vi "http 400 bad request.vi"(11 "application request in":T4) -> (3 "application request out":T1)   [LabVIEW 2016, in "Basic HTTP server.lvclass"]
uses:
  Basic HTTP server.lvclass
  http request.ctl
  http method.ctl
  HTTP headers/http header data.ctl
  http response.ctl
  http response packet type.ctl
  HTTP headers/http headers.lvlib
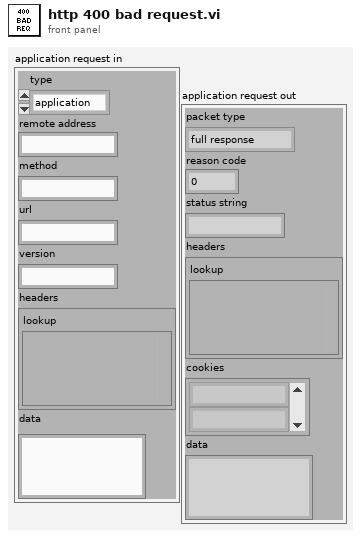
[diagram p1: front panel]
types:
  T1 = typedef "Basic HTTP server.lvclass/http response.ctl" = cluster{"packet type":T2, "reason code":u16, "status string":string, "headers":T3, "cookies":string[], "data":string}
  T2 = typedef "Basic HTTP server.lvclass/http response packet type.ctl" = enum16{"full response", "header only", "data only", "last data", "raw output"}
  T3 = typedef "http headers.lvlib/http header data.ctl" = cluster{"lookup":variant}
  T4 = typedef "Basic HTTP server.lvclass/http request.ctl" = cluster{"type":T5, "remote address":string, "method":string, "url":string, "version":string, "headers":T3, "data":string}
  T5 = typedef "Basic HTTP server.lvclass/http method.ctl" = enum16{"application", "error", "upgrade", "expect"}
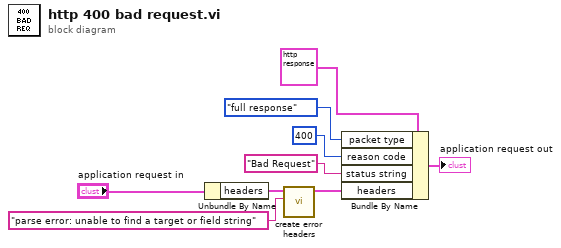
[diagram p0: block diagram]
diagram:
  n1 = Unbundle By Name("application request in") -> ("headers"=w1:T3)
  n2 = call "create error headers.vi"("custom error reason"="parse error: unable to find a target or field string" ("name"), "headers in"=w1) -> ("headers out"=w2:T3)  [unwired: 9 in]
  n3 = Bundle By Name(cluster=T1 {"packet type"=enum."full response", "reason code"=0, "status string"="", "headers"={"lookup"=variant}, "cookies"=[], "data"=""} ("application request"), "packet type"=http_response_packet_type."full response", "reason code"=u16 400, "status string"="Bad Request", "headers"=w2) -> (→"application request out":T1)
